vi "Anayze SPR curve.vi"(10 "New intensity arr":dbl[](array[numeric]), 11 "New angle arr":dbl[](array[numeric])) -> (3 "Cluster":T1 {"Curve width" format="%#.3g°"; "Maximum Intensity" format="%#_gV"; "q Middle" format="%#_g°"; "Minimum Intensity" format="%#_gV"; "qR" format="%#_g°"})   [LabVIEW 2020]
uses:
  controls/Analysis results -- cluster.ctl
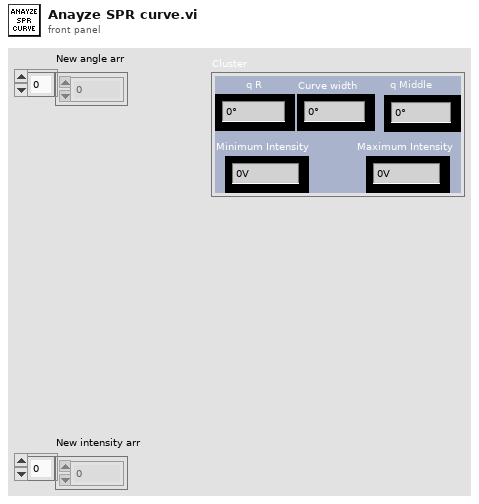
[diagram p1: front panel]
types:
  T1 = typedef "Analysis results -- cluster.ctl" = cluster{"q Middle":dbl, "Curve width":dbl, "Maximum Intensity":dbl, "Minimum Intensity":dbl, "qR ":dbl}
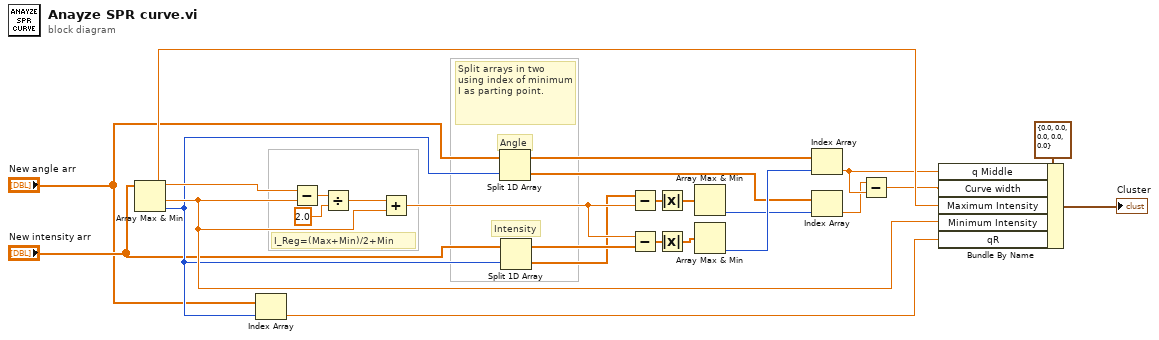
[diagram p0: block diagram]
diagram:
  # "Intensity"
  # "Angle"
  # "Split arrays in two using index of minimum I as parting point."
  # "I_Reg=(Max+Min)/2+Min"
  n1 = Array Max & Min(array="New intensity arr") -> (max value=w22:dbl, min value=w23:dbl, min index (indices)=w8:i32)  [unwired: 1 out]
  n2 = Index Array(array="New angle arr", index=w8) -> (element=w24:dbl)
  n3 = Subtract(x=w22, y=w23) -> (x-y=w16:dbl)
  n4 = Divide(x=w16, y=2.0) -> (x/y=w14:dbl)
  n5 = Add(x=w14, y=w23) -> (x+y=w17:dbl)
  n6 = Split 1D Array(array="New angle arr", index=w8) -> (first subarray=w11:dbl[], second subarray=w9:dbl[])
  n7 = Split 1D Array(array="New intensity arr", index=w8) -> (first subarray=w18:dbl[], second subarray=w5:dbl[])
  n8 = Subtract(x=w5, y=w17) -> (x-y=w6:dbl[])
  n9 = Subtract(x=w17, y=w18) -> (x-y=w13:dbl[])
  n10 = Absolute Value(x=w6) -> (abs(x)=w7:dbl[])
  n11 = Absolute Value(x=w13) -> (abs(x)=w12:dbl[])
  n12 = Array Max & Min(array=w7) -> (min index (indices)=w4:i32)  [unwired: 3 out]
  n13 = Array Max & Min(array=w12) -> (min index (indices)=w10:i32)  [unwired: 3 out]
  n14 = Index Array(array=w11, index=w10) -> (element=w20:dbl)
  n15 = Index Array(array=w9, index=w4) -> (element=w3:dbl)
  n16 = Subtract(x=w3, y=w20) -> (x-y=w21:dbl)
  n17 = Bundle By Name(cluster=T1 {"q Middle"=0.0, "Curve width"=0.0, "Maximum Intensity"=0.0, "Minimum Intensity"=0.0, "qR "=0.0} ("Cluster"), "q Middle"=w20, "Curve width"=w21, "Maximum Intensity"=w22, "Minimum Intensity"=w23, "qR"=w24) -> (→"Cluster":T1)
